vi "Handle Message.vi"(7 "priority":T1, 8 "error in (no error)":errorcluster, 10 "Message":refnum<class "Message.lvclass">, 11 "AF MQTT Message Channel in":refnum<class "AF MQTT Message Channel.lvclass">) -> (0 "error out":errorcluster)   [LabVIEW 2020, in "AF MQTT Channel.lvlib" / "AF MQTT Message Channel.lvclass"]
uses:
  AF MQTT Message Channel.lvclass
  AF MQTT Message Channel.lvclass/AF MQTT Message Channel.ctl
  <vilib>/LabVIEW Open Source Project/MQTT Client/Client class/Client.lvclass
  <vilib>/ActorFramework/Message Dequeuer/Dequeue Priority.ctl
  <vilib>/ActorFramework/Message Dequeuer/Message Dequeuer.lvclass
  <vilib>/ActorFramework/Message/Message.lvclass
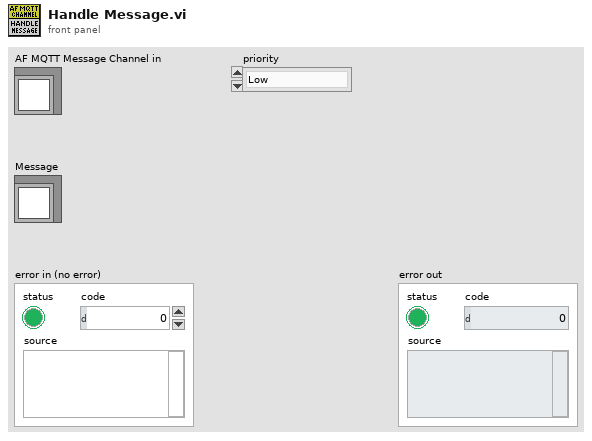
[diagram p1: front panel]
types:
  T1 = typedef "Actor Framework.lvlib/Message Dequeuer.lvclass/Dequeue Priority.ctl" = enum16{"Low", "Normal", "High", "Critical"}
  T2 = typedef "MQTT_Control_Packets.lvlib/ControlPacket.lvclass/QualityOfService -- enum.ctl" = enum16{"0 (At Most Once)", "1 (At Least Once)", "2 (Exactly Once)"}
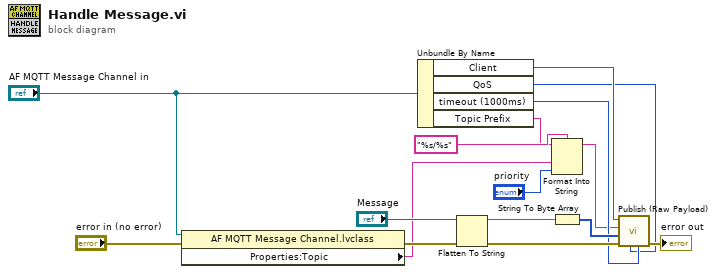
[diagram p0: block diagram]
diagram:
  n1 = property class="AF MQTT Message Channel.lvclass"(reference="AF MQTT Message Channel in", error in="error in (no error)") -> (error out=w15:errorcluster, "Properties:Topic"=w4:string)  [unwired: 1 out]
  n2 = Unbundle By Name("AF MQTT Message Channel in") -> ("Client"=w14:refnum<class "Client.lvclass">, "QoS"=w7:T2, "timeout (1000ms)"=w8:i32, "Topic Prefix"=w1:string)
  n3 = Flatten To String(anything="Message", error in (no error)=w15) -> (data string=w13:string, error out=w10:errorcluster)  [unwired: 2 in, 1 out]
  n4 = Format Into String(format string="%s/%s", initial string=w1, w4, "priority") -> (resulting string=w2:string)  [unwired: 1 in, 1 out]
  n5 = String To Byte Array(string=w13) -> (unsigned byte array=w12:u8[])
  n6 = call <vilib>:"Publish (Raw Payload).vi"("timeout (1000ms)"=w8, "QoS"=w7, "error in (no error)"=w10, "Binary Payload"=w12, "Topic Name"=w2, "Client in"=w14) -> ("error out"=→"error out":errorcluster)  [unwired: 3 in, 2 out]
